vi "Determine Distance to Tags.vi"(6 "error in (no error)":errorcluster, 7 "Error Margin":dbl=2.0, 8 "Enable Error margin?":bool, 9 "Input TagsArray":refnum<class "Tag.lvclass">[](array[class]), 10 "Input Tag.lvclass":refnum<class "Tag.lvclass">, 11 "DistanceLimitTag":dbl=70.0) -> (2 "TagDistanceArray":T1(array[cluster]), 4 "error out":errorcluster)   [LabVIEW 2014, in "Tag.lvclass"]
uses:
  Tag.lvclass
panel:
  out "From Tag":refnum<class "Tag.lvclass">
  out "To Tag":refnum<class "Tag.lvclass">
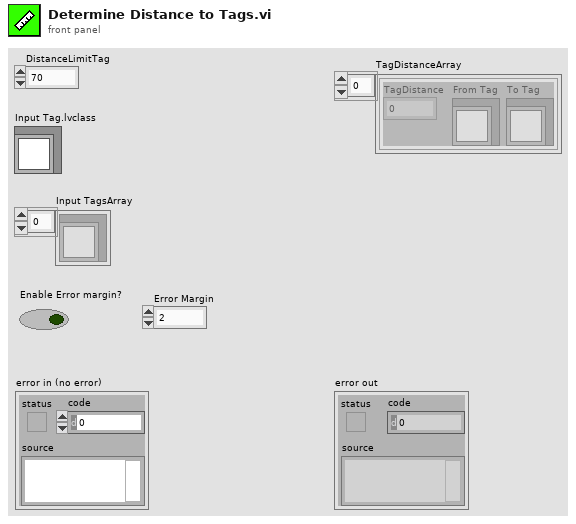
[diagram p1: front panel]
types:
  T1 = cluster{"TagDistance":dbl, "From Tag":refnum<class "Tag.lvclass">, "To Tag":refnum<class "Tag.lvclass">}[]
  T2 = cluster{dbl, "From Tag":refnum<class "Tag.lvclass">, "To Tag":refnum<class "Tag.lvclass">}
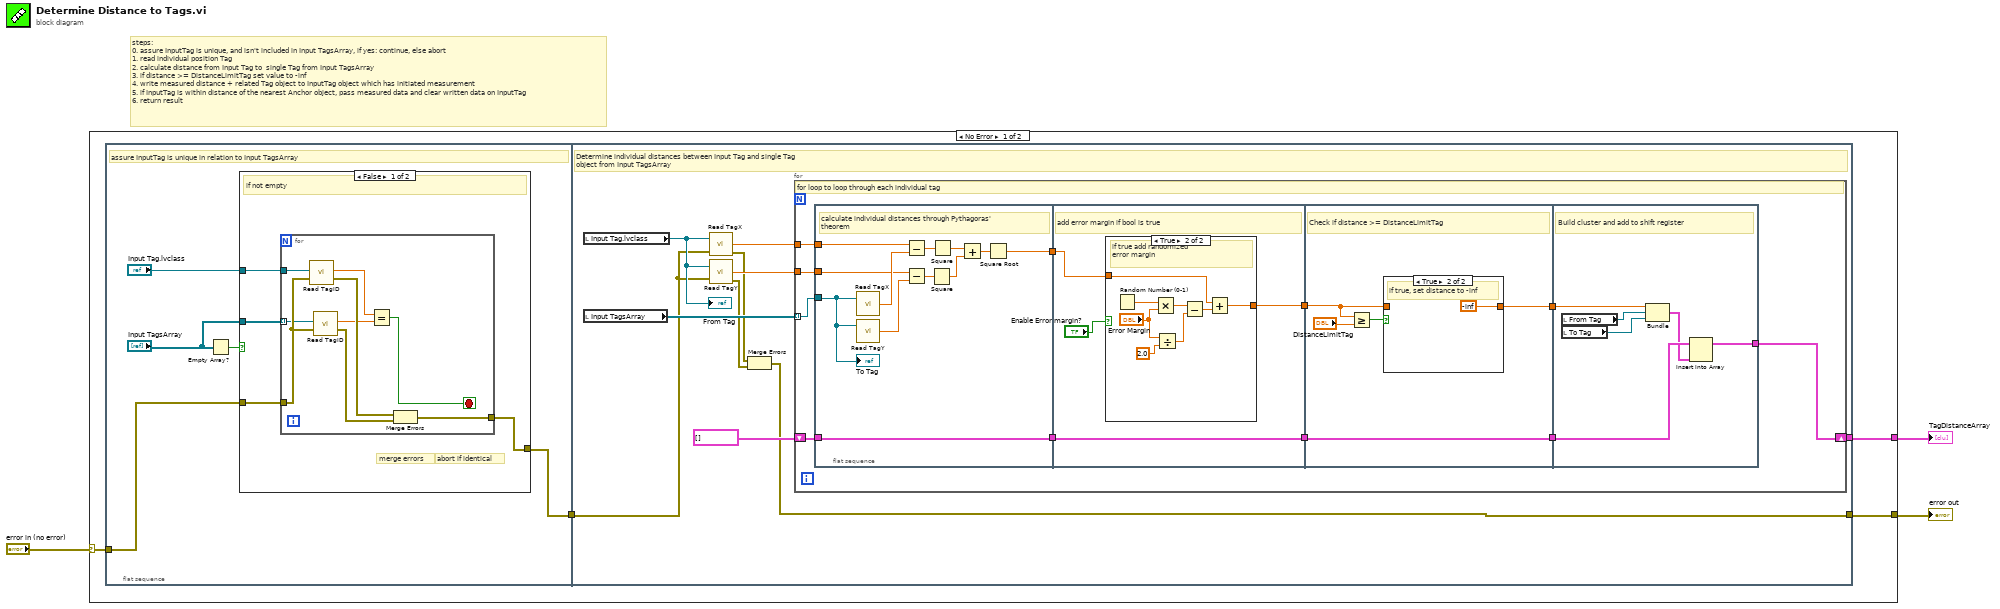
[diagram p0: block diagram]
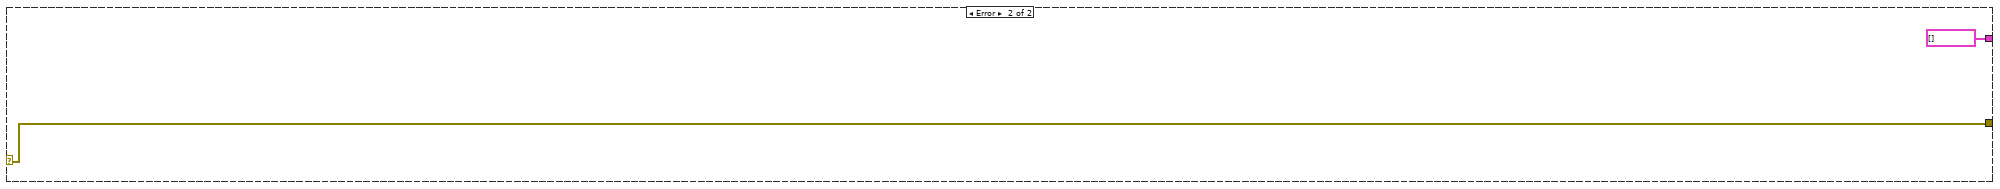
[diagram p5: hidden frame]
diagram:
  # "steps: \n0. assure InputTag is unique, and isn't included in Input TagsArray, if yes: continue, else abort\n1. read individual position Tag\n2. calculate distance from Input Tag to  single Tag from Input TagsArray\n3. if distance >= DistanceLimitTag set value to -inf\n4. write measured distance + related Tag object to InputTag object which has initiated measurement\n5. if InputTag is within distance of the nearest Anchor object, pass measured data and clear written data on InputTag\n6. return result"
  n1 = case shown="No Error" "error in (no error)" {
    selector: "error in (no error)" -> [w7 w87]
    tunnel: [w6 w87] -> w2
    tunnel: [w4 T1 [] ("TagDistanceArray")] -> w1
    frame No Error {
      n2 = flat-sequence {
        tunnel: w7 -> [w10]
        tunnel: [w9] -> w5
        tunnel: [w27] -> w6
        tunnel: w5 -> [w30]
        tunnel: [w31] -> w4
        frame #0 {
          # "assure InputTag is unique in relation to Input TagsArray"
          n3 = Empty Array?(array="Input TagsArray") -> (empty?=w12:bool)
          n4 = case shown="False" w12 {
            tunnel: "Input TagsArray" -> [w16 _]
            tunnel: w10 -> [w15 w26]
            tunnel: [w14 w26] -> w9
            tunnel: "Input Tag.lvclass" -> [w13 _]
            frame False {
              # "abort if identical"
              # "merge errors"
              # "if not empty"
              n5 = for {
                tunnel: w16 -> [w17] mode=indexing
                tunnel: w15 -> [w21]
                tunnel: [w25] -> w14
                tunnel: w13 -> [w23]
                stop <- w24 stop-if-true
                n6 = call "Read TagID.vi"("Tag in"=w23, "error in (no error)"=w21) -> ("TagID"=w20:dbl, "error out"=w22:errorcluster)  [unwired: 15 in, 1 out]
                n7 = call "Read TagID.vi"("Tag in"=w17, "error in (no error)"=w21) -> ("TagID"=w19:dbl, "error out"=w18:errorcluster)  [unwired: 15 in, 1 out]
                n8 = Equal?(x=w20, y=w19) -> (x = y?=w24:bool)
                n9 = Merge Errors(w22, w18) -> (w25:errorcluster)
              }
            }
            frame True {
              # "if empty"
            }
          }
        }
        frame #1 {
          # "Determine individual distances between Input Tag and single Tag\nobject from Input TagsArray"
          n10 = local read "Input Tag.lvclass"() -> (w36:refnum<class "Tag.lvclass">)
          "From Tag" <- w36
          n11 = local read "Input TagsArray"() -> (w35:refnum<class "Tag.lvclass">[])
          n12 = call-dynamic "Read TagX.vi"("Tag in"=w36, "error in (no error)"=w30) -> ("RealTagX"=w33:dbl, "error out"=w28:errorcluster)  [unwired: 1 out]
          n13 = call-dynamic "Read TagY.vi"("Tag in"=w36, "error in (no error)"=w30) -> ("RealTagY"=w34:dbl, "error out"=w29:errorcluster)  [unwired: 1 out]
          n14 = Merge Errors(w28, w29) -> (w27:errorcluster)
          n15 = for {
            tunnel: w35 -> [w47] mode=indexing
            tunnel: w34 -> [w45]
            tunnel: w33 -> [w46]
            shift-right: [w41] -> w31
            shift-left: T1 [] ("TagDistanceArray") -> [w42]
            # "for loop to loop through each individual tag"
            n16 = flat-sequence {
              tunnel: w47 -> [w59]
              tunnel: w46 -> [w58]
              tunnel: w45 -> [w56]
              tunnel: [w49] -> w44
              tunnel: [w48] -> w43
              tunnel: w42 -> [w48]
              tunnel: w44 -> [w62]
              tunnel: w43 -> [w61]
              tunnel: [w61] -> w40
              tunnel: [w60] -> w38
              tunnel: w40 -> [w77]
              tunnel: [w77] -> w39
              tunnel: w38 -> [w74]
              tunnel: [w73] -> w37
              tunnel: w39 -> [w82]
              tunnel: w37 -> [w85]
              tunnel: [w80] -> w41
              frame #0 {
                # "calculate individual distances through Pythagoras'\ntheorem"
                n17 = call-dynamic "Read TagX.vi"("Tag in"=w59) -> ("RealTagX"=w57:dbl)  [unwired: 1 in, 2 out]
                n18 = call-dynamic "Read TagY.vi"("Tag in"=w59) -> ("RealTagY"=w55:dbl)  [unwired: 1 in, 2 out]
                n19 = Subtract(x=w58, y=w57) -> (x-y=w54:dbl)
                n20 = Subtract(x=w56, y=w55) -> (x-y=w53:dbl)
                n21 = Square(x=w53) -> (x^2=w51:dbl)
                n22 = Square(x=w54) -> (x^2=w52:dbl)
                n23 = Add(x=w52, y=w51) -> (x+y=w50:dbl)
                n24 = Square Root(x=w50) -> (sqrt(x)=w49:dbl)
                "To Tag" <- w59
              }
              frame #1 {
                # "add error margin if bool is true"
                n25 = case shown="True" "Enable Error margin?" {
                  tunnel: w62 -> [w64 w66]
                  tunnel: [w64 w65] -> w60
                  frame False {
                  }
                  frame True {
                    # "if true add randomized \nerror margin"
                    n26 = Random Number (0-1)() -> (number: 0 to 1=w72:dbl)
                    n27 = Multiply(x=w72, y="Error Margin") -> (x*y=w69:dbl)
                    n28 = Divide(x="Error Margin", y=2.0) -> (x/y=w68:dbl)
                    n29 = Subtract(x=w69, y=w68) -> (x-y=w67:dbl)
                    n30 = Add(x=w66, y=w67) -> (x+y=w65:dbl)
                  }
                }
              }
              frame #2 {
                # "Check if distance >= DistanceLimitTag"
                n31 = Greater Or Equal?(x=w74, y="DistanceLimitTag") -> (x >= y?=w75:bool)
                n32 = case shown="True" w75 {
                  tunnel: w74 -> [w78 _]
                  tunnel: [w78 -inf] -> w73
                  frame False {
                  }
                  frame True {
                    # "if true, set distance to -inf"
                  }
                }
              }
              frame #3 {
                # "Build cluster and add to shift register"
                n33 = local read "From Tag"() -> (w84:refnum<class "Tag.lvclass">)
                n34 = local read "To Tag"() -> (w83:refnum<class "Tag.lvclass">)
                n35 = Bundle(w85, "From Tag"=w84, "To Tag"=w83) -> (w81:T2)  [unwired: 1 in]
                n36 = Insert Into Array(array=w82, new element=w81) -> (w80:T1)  [unwired: 1 in]
              }
            }
          }
        }
      }
    }
    frame Error {
    }
  }
  "error out" <- w2
  "TagDistanceArray" <- w1
